vi "PrimeAndResetConditions.vi"(8 "error in (no error)":errorcluster, 10 "conditions in":T1[](array[typedef])=[{"Condition"={"Source"="", "Type"="", "Operator"="", "CompareTo"="", "DwellSeconds"=0.0}, "LatchValue"="", "LatchTime"=timestamp(0 s since 1904-01-01)}, {"Condition"={"Source"="", "Type"="", "Operator"="", "CompareTo"="", "DwellSeconds"=0.0}, "LatchValue"="", "LatchTime"=timestamp(0 s since 1904-01-01)}], 11 "SnapshotMap":T3) -> (0 "error out":errorcluster, 2 "conditions out":T1[](array[typedef]))   [LabVIEW 2017, in "Trigger.lvlib"]
uses:
  <vilib>/addons/InsightCM/Devices/Shared/Common/Trigger/Trigger.lvlib
  <vilib>/addons/InsightCM/Devices/Shared/Common/Trigger/controls/TriggerCondition.ctl
  <vilib>/addons/InsightCM/MessageBus/Base/controls/Condition.ctl
  <vilib>/addons/PointValueMap/controls/PointMap.ctl
  <vilib>/addons/PointValueMap/PointValueMap.lvlib
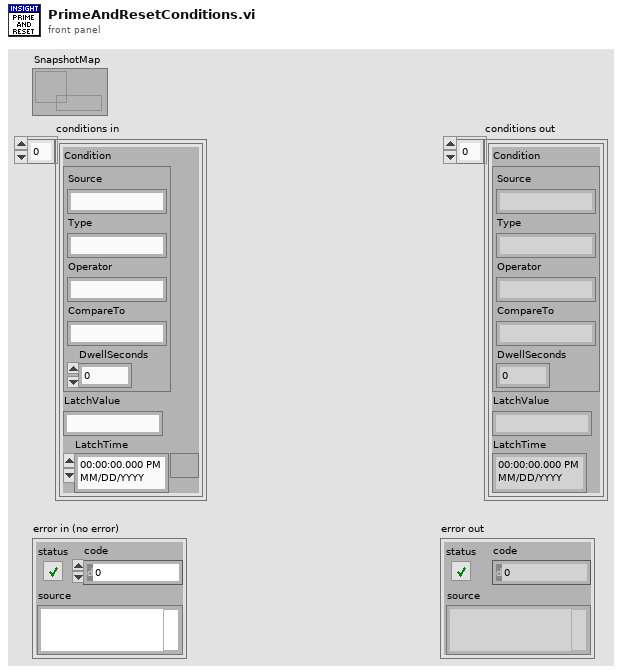
[diagram p1: front panel]
types:
  T1 = typedef "Trigger.lvlib/TriggerCondition.ctl" = cluster{"Condition":T2, "LatchValue":string, "LatchTime":timestamp}
  T2 = typedef "Condition.ctl" = cluster{"Source":string, "Type":string, "Operator":string, "CompareTo":string, "DwellSeconds":dbl}
  T3 = typedef "PointValueMap.lvlib/PointMap.ctl" = refnum<data-value>
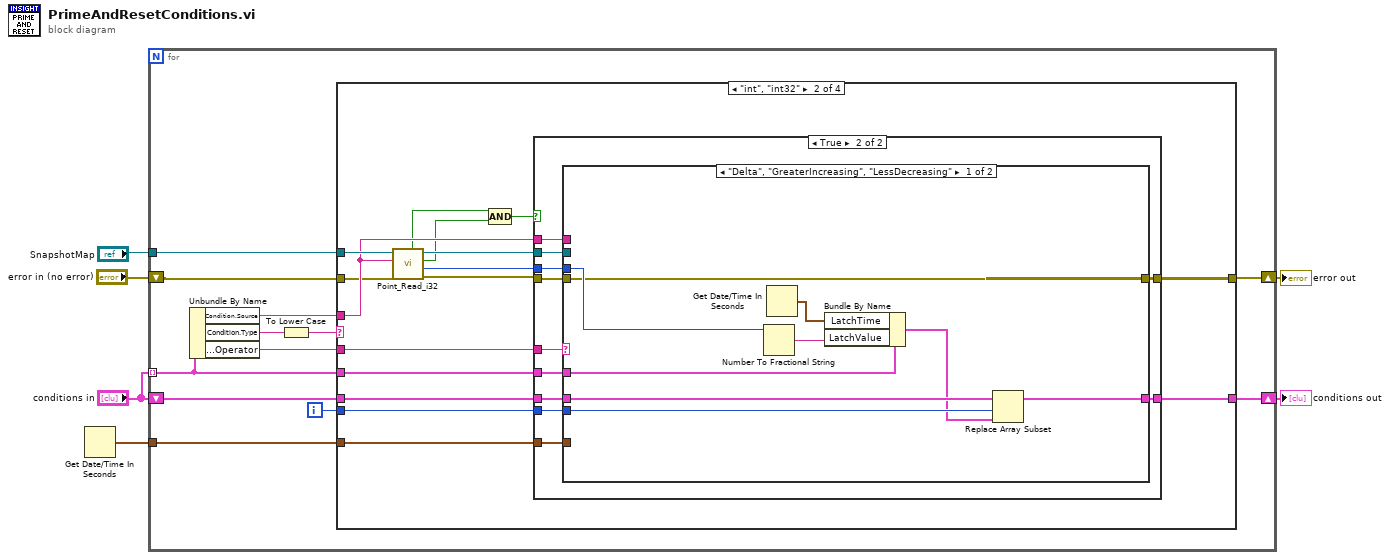
[diagram p0: block diagram]
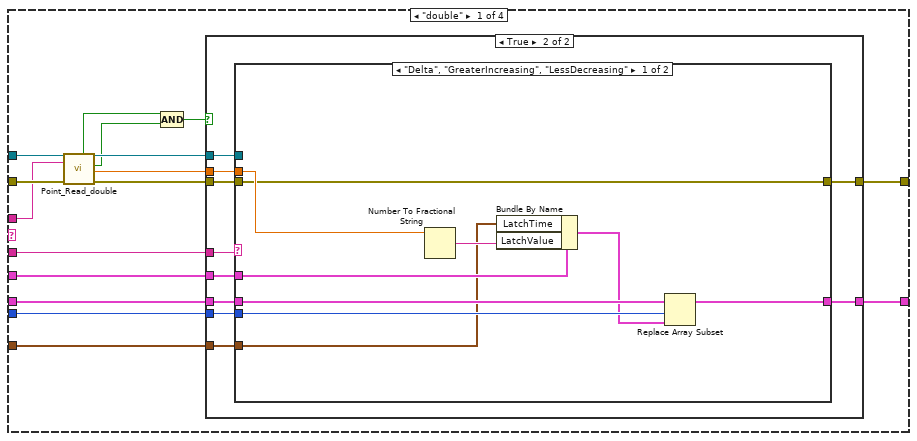
[diagram p2: hidden frame]
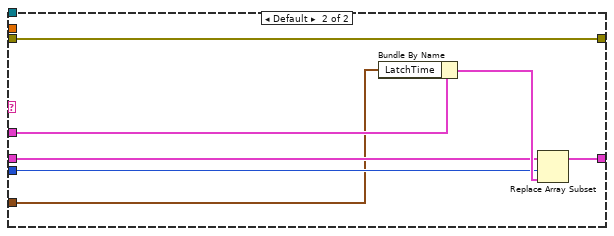
[diagram p4: hidden frame]
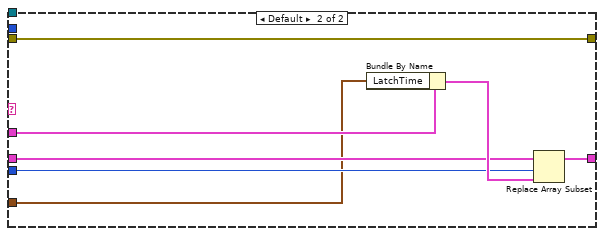
[diagram p6: hidden frame]
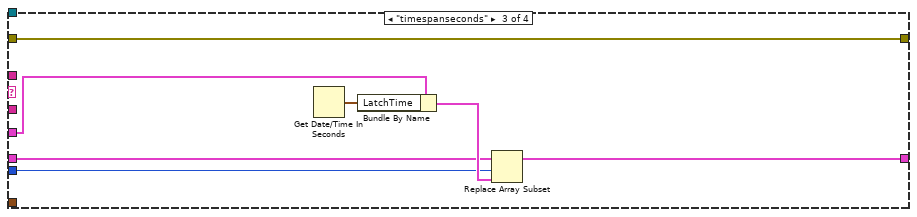
[diagram p7: hidden frame]
diagram:
  n1 = Get Date/Time In Seconds() -> (seconds since 1Jan1904=w1:timestamp)
  n2 = for {
    tunnel: "conditions in" -> [w11] mode=indexing
    tunnel: "SnapshotMap" -> [w15]
    shift-right: [w12] -> w4
    shift-left: "error in (no error)" -> [w14]
    shift-right: [w8] -> w2
    shift-left: "conditions in" -> [w9]
    tunnel: w1 -> [w7]
    i -> [w10]
    n3 = Unbundle By Name(w11) -> ("Condition.Source"=w13:string, "Condition.Type"=w18:string, "Condition.Operator"=w17:string)
    n4 = To Lower Case(string=w18) -> (all lower case string=w16:string)
    n5 = case shown="\"int\", \"int32\"" w16 {
      tunnel: w17 -> [w31 w77 _ _]
      tunnel: w15 -> [w34 w71 _ _]
      tunnel: w13 -> [w30 w69 _ _]
      tunnel: w14 -> [w33 w68 w109 w115]
      tunnel: [w32 w78 w109 w115] -> w12
      tunnel: w11 -> [w28 w76 w110 _]
      tunnel: w10 -> [w27 w75 w111 _]
      tunnel: w9 -> [w26 w74 w113 w116]
      tunnel: [w25 w73 w112 w116] -> w8
      tunnel: w7 -> [w19 w63 _ _]
      frame "double" {
        n6 = call <vilib>:"Point_Read_double.vi"("Error In"=w33, "Tag"=w30, "Map"=w34) -> ("Error Out"=w20:errorcluster, "Value"=w24:dbl, "Found?"=w23:bool, "Map Out"=w29:T3, "Valid?"=w22:bool)  [unwired: 3 in, 1 out]
        n7 = Compound Arithmetic op=AND(w22, w23) -> (w21:bool)
        n8 = case shown="True" w21 {
          tunnel: [w36 w46] -> w32
          tunnel: w31 -> [_ w45]
          tunnel: w29 -> [_ w44]
          tunnel: w20 -> [w36 w43]
          tunnel: w28 -> [_ w42]
          tunnel: w27 -> [_ w41]
          tunnel: w26 -> [w35 w40]
          tunnel: [w35 w39] -> w25
          tunnel: w24 -> [_ w38]
          tunnel: w19 -> [_ w37]
          frame False {
            # "Source or compare to tag not valid or found in PVM"
          }
          frame True {
            n9 = case shown="\"Delta\", \"GreaterIncreasing\", \"LessDecreasing\"" w45 {
              tunnel: w38 -> [w51 _]
              tunnel: w43 -> [w50 w58]
              tunnel: [w50 w58] -> w46
              tunnel: w44 -> [_ _]
              tunnel: w42 -> [w55 w60]
              tunnel: w41 -> [w52 w59]
              tunnel: w40 -> [w54 w61]
              tunnel: [w53 w57] -> w39
              tunnel: w37 -> [w47 w56]
              frame "Delta", "GreaterIncreasing", "LessDecreasing" {
                n10 = Number To Fractional String(number=w51) -> (F-format string=w49:string)  [unwired: 3 in]
                n11 = Bundle By Name(cluster=w55, "LatchTime"=w47, "LatchValue"=w49) -> (w48:T1)
                n12 = Replace Array Subset(array=w54, new element=w48, index=w52) -> (w53:T1[])
              }
              frame Default {
                n13 = Bundle By Name(cluster=w60, "LatchTime"=w56) -> (w62:T1)
                n14 = Replace Array Subset(array=w61, new element=w62, index=w59) -> (w57:T1[])
              }
            }
          }
        }
      }
      frame "int", "int32" {
        n15 = call <vilib>:"Point_Read_i32.vi"("Error In"=w68, "Tag"=w69, "Map"=w71) -> ("Error Out"=w64:errorcluster, "Value"=w65:i32, "Found?"=w66:bool, "Map Out"=w70:T3, "Valid?"=w67:bool)  [unwired: 3 in, 1 out]
        n16 = Compound Arithmetic op=AND(w67, w66) -> (w72:bool)
        n17 = case shown="True" w72 {
          tunnel: [w80 w91] -> w78
          tunnel: w77 -> [_ w90]
          tunnel: w69 -> [_ w89]
          tunnel: w70 -> [_ w88]
          tunnel: w64 -> [w80 w87]
          tunnel: w76 -> [_ w86]
          tunnel: w75 -> [_ w85]
          tunnel: w74 -> [w79 w84]
          tunnel: [w79 w83] -> w73
          tunnel: w65 -> [_ w82]
          tunnel: w63 -> [_ w81]
          frame False {
          }
          frame True {
            n18 = case shown="\"Delta\", \"GreaterIncreasing\", \"LessDecreasing\"" w90 {
              tunnel: w82 -> [w96 _]
              tunnel: w87 -> [w95 w104]
              tunnel: [w95 w104] -> w91
              tunnel: w88 -> [_ _]
              tunnel: w89 -> [_ _]
              tunnel: w86 -> [w100 w103]
              tunnel: w85 -> [w97 w105]
              tunnel: w84 -> [w99 w106]
              tunnel: [w98 w102] -> w83
              tunnel: w81 -> [_ w101]
              frame "Delta", "GreaterIncreasing", "LessDecreasing" {
                n19 = Number To Fractional String(number=w96) -> (F-format string=w94:string)  [unwired: 3 in]
                n20 = Get Date/Time In Seconds() -> (seconds since 1Jan1904=w92:timestamp)
                n21 = Bundle By Name(cluster=w100, "LatchTime"=w92, "LatchValue"=w94) -> (w93:T1)
                n22 = Replace Array Subset(array=w99, new element=w93, index=w97) -> (w98:T1[])
              }
              frame Default {
                n23 = Bundle By Name(cluster=w103, "LatchTime"=w101) -> (w107:T1)
                n24 = Replace Array Subset(array=w106, new element=w107, index=w105) -> (w102:T1[])
              }
            }
          }
        }
      }
      frame "timespanseconds" {
        n25 = Get Date/Time In Seconds() -> (seconds since 1Jan1904=w108:timestamp)
        n26 = Bundle By Name(cluster=w110, "LatchTime"=w108) -> (w114:T1)
        n27 = Replace Array Subset(array=w113, new element=w114, index=w111) -> (w112:T1[])
      }
      frame Default {
      }
    }
  }
  "error out" <- w4
  "conditions out" <- w2
